vi "Parse Array of Bytes (uSMC).vi"(0 "byte array":u8[](array[numeric])) -> (1 "first 2 bytes":u16, 2 "second 2 bytes":u16, 3 "array buffer":u8[](array[numeric]))   [LabVIEW 2010, in "SignalWriterMH110203USBStepperMotor.lvclass"]
uses:
  SignalWriterMH110203USBStepperMotor.lvclass
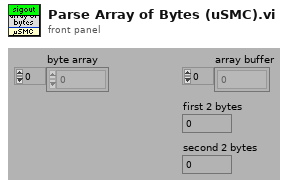
[diagram p1: front panel]
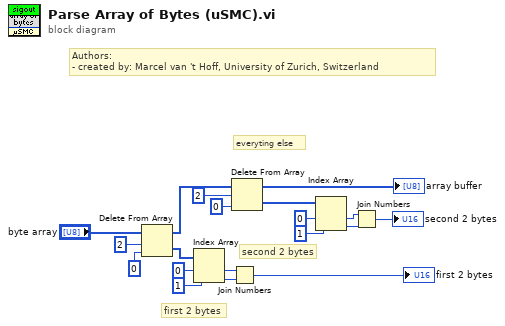
[diagram p0: block diagram]
diagram:
  # "Authors: \n- created by: Marcel van 't Hoff, University of Zurich, Switzerland"
  # "everyting else"
  # "second 2 bytes"
  # "first 2 bytes"
  n1 = Delete From Array(array="byte array", length=2, index=0) -> (deleted portion=w13:u8[], array with subset deleted=w15:u8[])
  n2 = Index Array(array=w13, index #1=0 ("index"), index #2=1 ("index")) -> (element #1=w9:u8, element #2=w10:u8)
  n3 = Join Numbers(hi=w9, lo=w10) -> ((hi.lo)=→"first 2 bytes":u16)
  n4 = Delete From Array(array=w15, length=2, index=0) -> (deleted portion=w4:u8[], array with subset deleted=→"array buffer":u8[])
  n5 = Index Array(array=w4, index #1=0 ("index"), index #2=1 ("index")) -> (element #1=w8:u8, element #2=w7:u8)
  n6 = Join Numbers(hi=w8, lo=w7) -> ((hi.lo)=→"second 2 bytes":u16)
